vi "Actor Core.vi"(8 "error in":errorcluster, 11 "server in":refnum<class "server.lvclass">) -> (0 "error out":errorcluster, 3 "Actor out":refnum<class "Actor.lvclass">)   [LabVIEW 2016, in "server.lvlib" / "server.lvclass"]
doc: "(<B>Filename</B>: Actor Framework.lvlib:Actor.lvclass:Actor Core.vi)\n\nReceives messages to the actor, reacts to them, and initiates any error handling that may shut the actor down.\n\nDescendant classes may override this VI to append parallel tasks for the actor to complete while it handles messages. Overrides use the Call Parent Method node."
uses:
  server.lvclass
  C:/Program Files/National Instruments/LabVIEW 2016/vi.lib/ActorFramework/Actor/Actor.lvclass
  <vilib>/ActorFramework/Actor/Actor.lvclass
  <vilib>/ActorFramework/Message Enqueuer/Message Enqueuer.lvclass
  server.lvclass/server.ctl
  <vilib>/ActorFramework/Actor/Actor.lvclass/Actor.ctl
  <vilib>/ActorFramework/Message Enqueuer/Message Enqueuer.lvclass/Message Enqueuer.ctl
  client/client/client.lvclass
  <vilib>/ActorFramework/Message Enqueuer/Init from Existing Queue.vi
  <vilib>/ActorFramework/Message Enqueuer/Enqueue.vi
  <vilib>/ActorFramework/Stop Msg/Stop Msg.lvclass
  C:/Program Files/National Instruments/LabVIEW 2016/vi.lib/ActorFramework/Message/Message.lvclass
  <vilib>/ActorFramework/Message Priority Queue/Priority Enqueue.vi
panel:
  in  "stop":bool
  out "client number":i32
  in  "close client":bool
  in  "open client":bool
  out "DataRecord":string
  out "loop index":i32
  # "Server"
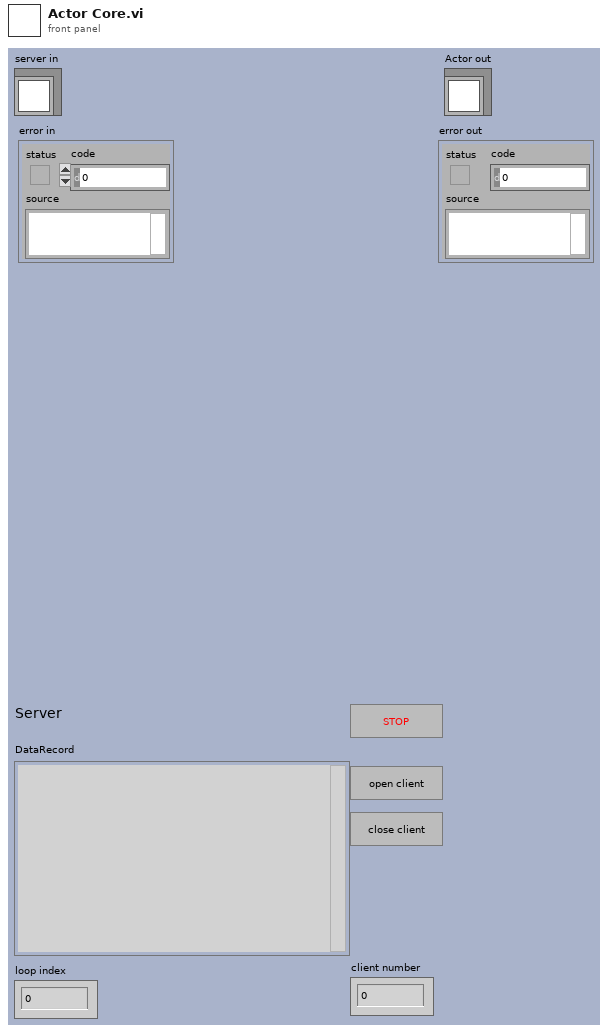
[diagram p1: front panel]
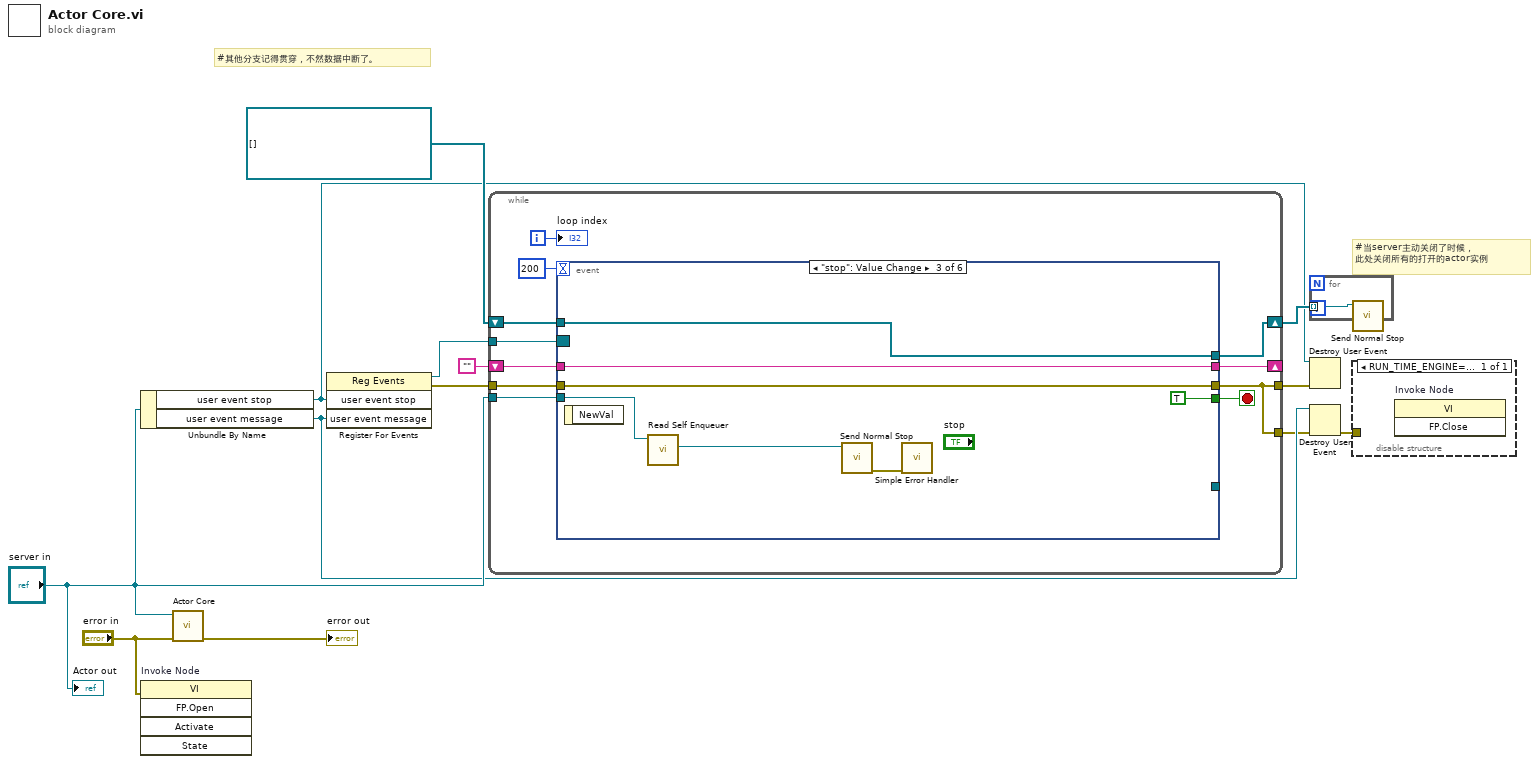
[diagram p0: block diagram]
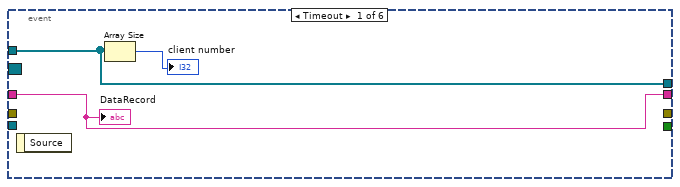
[diagram p2: hidden frame]
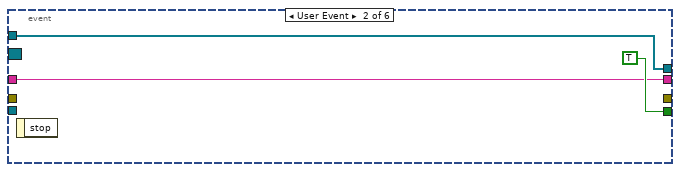
[diagram p3: hidden frame]
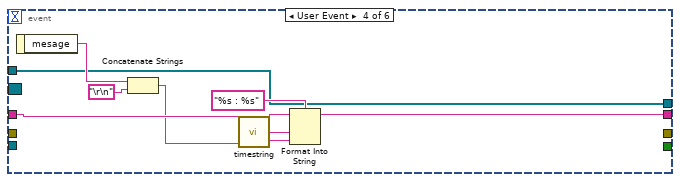
[diagram p4: hidden frame]
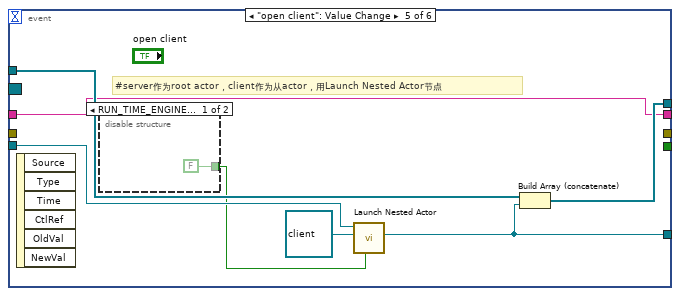
[diagram p5: hidden frame]
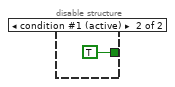
[diagram p6: hidden frame]
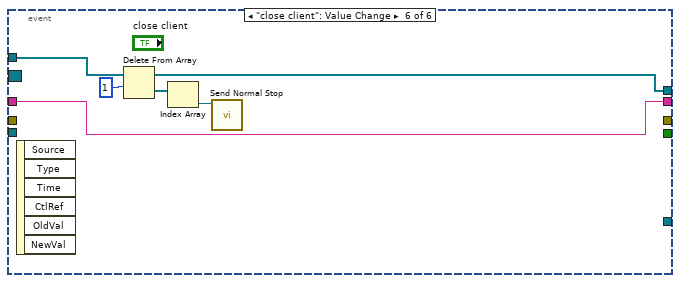
[diagram p7: hidden frame]
diagram:
  # "#其他分支记得贯穿，不然数据中断了。"
  # "#当server主动关闭了时候，\n此处关闭所有的打开的actor实例"
  n1 = Unbundle By Name("server in") -> ("user event stop"=w7:refnum<user-event>, "user event message"=w6:refnum<user-event>)
  n2 = invoke on="Invoke Node" class="VI" method="FP.Open"(error in="error in") -> ()  [unwired: 4 in, 5 out]
  n3 = call-parent "Actor Core.vi"("error in"="error in", "Actor in"="server in") -> ("error out"=→"error out":errorcluster)  [unwired: 8 in, 1 out]
  n4 = register-events(w7, w6) -> (reference out=w12:refnum<event-registration>, error out=w5:errorcluster)  [unwired: 2 in]
  n5 = while {
    tunnel: w12 -> [w24]
    shift-right: [w19] -> _
    shift-left: "" -> [w20]
    tunnel: "server in" -> [w18]
    shift-right: [w16] -> w9
    shift-left: refnum<class "Message Enqueuer.lvclass">[] [] ("Array") -> [w17]
    tunnel: w5 -> [w15]
    tunnel: [w14] -> w4
    tunnel: [w14] -> w3
    i -> [w22]
    stop <- w23 stop-if-true
    n6 = event shown="[2] \"stop\": Value Change" {
      selector: w24 -> [_ _ _ _ _ _]
      dyn-events: _ -> [_ _ _ _ _ _]
      timeout: 200 -> [_ _ _ _ _ _]
      tunnel: [_ TRUE TRUE _ _ _] -> w23
      tunnel: w20 -> [w27 w29 w36 w45 w47 w60]
      tunnel: [w27 w29 w36 w41 w47 w60] -> w19
      tunnel: w18 -> [_ _ w32 _ w52 _]
      tunnel: w17 -> [w26 w28 w35 w38 w50 w59]
      tunnel: [w26 w28 w35 w38 w49 w57] -> w16
      tunnel: [_ _ _ _ w46 _] -> _
      tunnel: [_ _ w33 _ _ _] -> w14
      tunnel: w15 -> [_ _ w33 _ _ _]
      event Timeout {
        n7 = event-data() -> ()  [unwired: 1 in, 1 out]
        n8 = Array Size(array=w26) -> (size(s)=→"client number":i32)
        "DataRecord" <- w27
      }
      event User Event {
        n9 = event-data() -> ()  [unwired: 1 in, 1 out]
      }
      event "stop": Value Change {
        n10 = event-data() -> ()  [unwired: 1 in, 1 out]
        n11 = call <vilib>:"Read Self Enqueuer.vi"("Actor"=w32) -> ("Self Enqueuer"=w34:refnum<class "Message Enqueuer.lvclass">)  [unwired: 10 in]
        n12 = call <vilib>:"Send Normal Stop.vi"("Message Enqueuer"=w34) -> ("error out"=w31:errorcluster)  [unwired: 10 in]
        n13 = call <vilib>:"Simple Error Handler.vi"("error in (no error)"=w31) -> ()  [unwired: 4 in, 5 out]
      }
      event User Event {
        n14 = event-data() -> ("mesage"=w43:string)  [unwired: 1 in]
        n15 = Concatenate Strings(w43, "\r\n") -> (w40:string)
        n16 = call "timestring.vi"() -> ("时间字符串"=w39:string)  [unwired: 5 in]
        n17 = Format Into String(format string="%s : %s" ("string"), initial string=w45, w39, w40) -> (resulting string=w41:string)  [unwired: 1 in, 1 out]
      }
      event "open client": Value Change {
        # "#server作为root actor，client作为从actor，用Launch Nested Actor节点"
        n18 = event-data() -> ()  [unwired: 1 in, 6 out]
        n19 = disable-structure shown="RUN_TIME_ENGINE==True" {
          disable-tunnel: [FALSE TRUE ("Open Actor Core front panel? (F)")] -> w48
          frame condition #0 {
          }
          frame condition #1 (active) {
          }
        }
        n20 = call <vilib>:"Launch Nested Actor.vi"("Open Actor Core front panel? (F)"=w48, "Nested Actor"=refnum<class "client.lvclass"> refnum ("client.lvlib:client.lvclass"), "Caller Actor in"=w52) -> ("Nested Actor's Enqueuer"=w46:refnum<class "Message Enqueuer.lvclass">)  [unwired: 6 in, 2 out]
        n21 = Build Array (concatenate)(w50, w46) -> (w49:refnum<class "Message Enqueuer.lvclass">[])
      }
      event "close client": Value Change {
        n22 = event-data() -> ()  [unwired: 1 in, 6 out]
        n23 = Delete From Array(array=w59, length=1) -> (deleted portion=w56:refnum<class "Message Enqueuer.lvclass">[], array with subset deleted=w57:refnum<class "Message Enqueuer.lvclass">[])  [unwired: 1 in]
        n24 = Index Array(array=w56) -> (element=w55:refnum<class "Message Enqueuer.lvclass">)  [unwired: 1 in]
        n25 = call <vilib>:"Send Normal Stop.vi"("Message Enqueuer"=w55) -> ()  [unwired: 10 in, 1 out]
      }
    }
    "loop index" <- w22
  }
  n26 = for {
    tunnel: w9 -> [w61] mode=indexing
    n27 = call <vilib>:"Send Normal Stop.vi"("Message Enqueuer"=w61) -> ()  [unwired: 10 in, 1 out]
  }
  n28 = Destroy User Event(user event=w7, error in=w4) -> ()  [unwired: 1 out]
  n29 = Destroy User Event(user event=w6, error in=w3) -> (error out=w2:errorcluster)
  n30 = disable-structure shown="RUN_TIME_ENGINE==True, Default" {
    disable-tunnel: w2 -> [_]
    frame condition #0 (active) {
      n31 = invoke on="Invoke Node" class="VI" method="FP.Close"() -> ()  [unwired: 3 in, 3 out]
    }
  }
  "Actor out" <- "server in"
